vi "colour pattern(SubVI).vi"() -> (0 "Color Selected":T1)   [LabVIEW 2020]
doc: "This VI randomly selects which color the game plays next."
uses:
  simon_colors.ctl
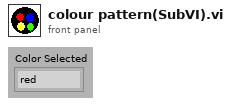
[diagram p1: front panel]
types:
  T1 = typedef "simon_colors.ctl" = enum16{"red", "green", "yellow", "blue"}
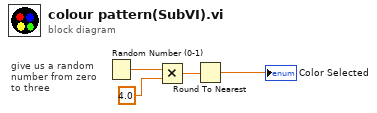
[diagram p0: block diagram]
diagram:
  # "give us a random\nnumber from zero\nto three"
  n1 = Random Number (0-1)() -> (number: 0 to 1=w3:dbl)
  n2 = Multiply(x=w3, y=4.0) -> (x*y=w2:dbl)
  n3 = Round To Nearest(number=w2) -> (nearest integer value=→"Color Selected":dbl)
